vi "GFITS_LibCreateImage.vi"(5 "amplifiers":u64, 6 "totkeys":i32, 7 "multiple extensions":bool, 8 "error in (no error)":errorcluster, 9 "hdutype":i32, 10 "datatype":i32, 11 "imname":string) -> (0 "error out":errorcluster, 2 "return value":u64, 3 "imname out":string)   [LabVIEW 2016]
uses:
  c/lib/libgfits.so
panel:
  in  "err":i32
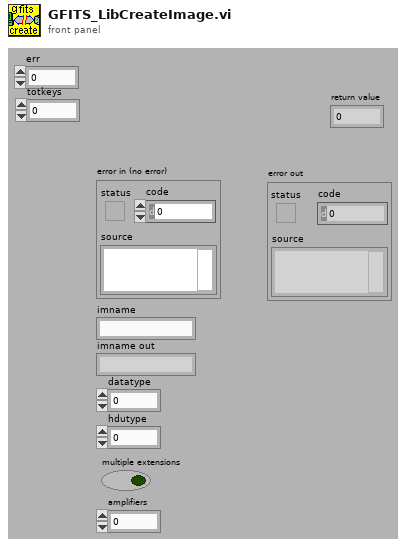
[diagram p1: front panel]
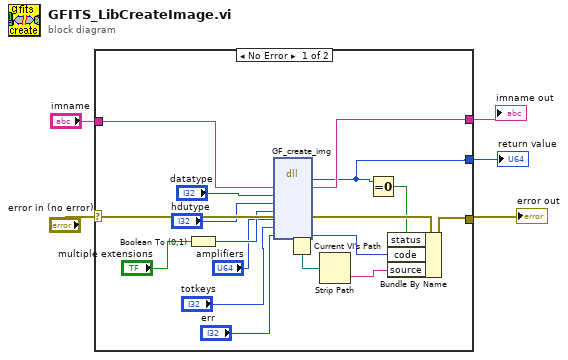
[diagram p0: block diagram]
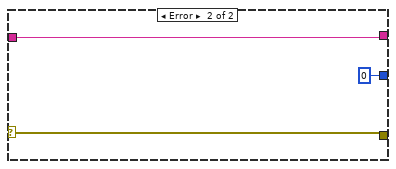
[diagram p2: hidden frame]
diagram:
  n1 = case shown="No Error" "error in (no error)" {
    selector: "error in (no error)" -> [w21 w24]
    tunnel: [w9 0] -> w5
    tunnel: [w17 w24] -> w3
    tunnel: "imname" -> [w16 w22]
    tunnel: [w15 w22] -> w1
    frame No Error {
      n2 = Boolean To (0,1)(Boolean="multiple extensions") -> (0, 1=w12:i16)
      n3 = dll-call lib="home/simager/panview/PAN/Modules/GFITS/private/c/lib/libgfits.so" fn="GF_create_img"("imname"=w16, "datatype"="datatype", "hdutype"="hdutype", "mult"=w12, "amplifiers"="amplifiers", "nkeys"="totkeys", "err"="err") -> ("return type"=w9:u64, "imname"=w15:string, "err"=w8:i32)  [unwired: 7 in, 3 out]
      n4 = Current VI's Path() -> (path=w19:path)
      n5 = Strip Path(path=w19) -> (name=w18:string)  [unwired: 1 out]
      n6 = Equal To 0?(x=w9) -> (x = 0?=w20:bool)
      n7 = Bundle By Name(cluster=w21, "status"=w20, "code"=w8, "source"=w18) -> (w17:errorcluster)
    }
    frame Error {
    }
  }
  "return value" <- w5
  "error out" <- w3
  "imname out" <- w1
